vi "ex_Change Control Caption.vi"(4 "error in (no error)":errorcluster, 5 "New Name":string, 6 "Old Name":string, 7 "VI refnum":refnum<vi>) -> (0 "error out":errorcluster, 3 "Ctl refnum out":refnum<vi>)   [LabVIEW 2020]
doc: "Changes the label and the caption for a control specified by the control refnum on the VI specified by the VI refnum."
panel:
  in  "Ctl refnum":refnum<vi>
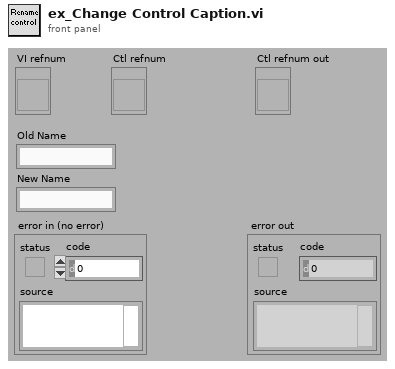
[diagram p1: front panel]
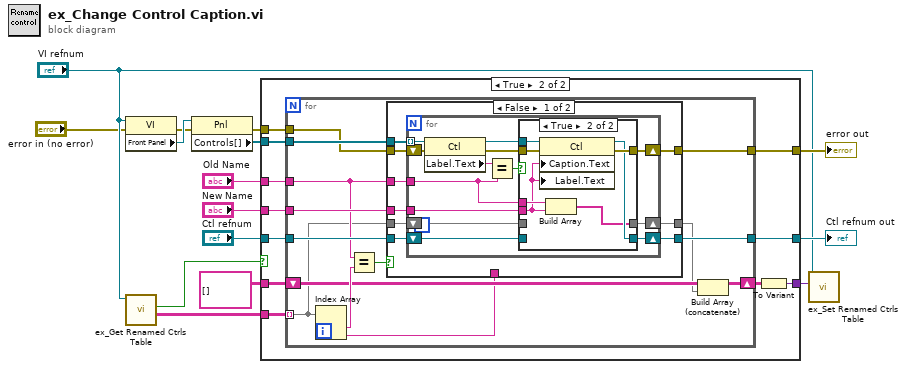
[diagram p0: block diagram]
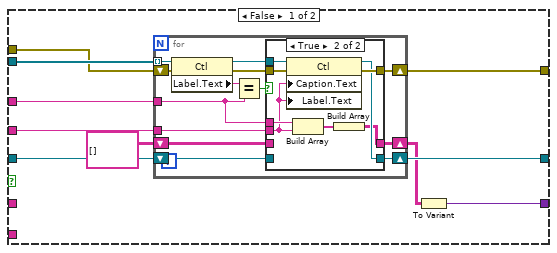
[diagram p2: hidden frame]
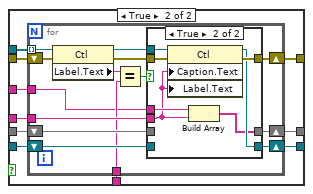
[diagram p5: hidden frame]
diagram:
  n1 = property class="VI"(reference="VI refnum", error in="error in (no error)") -> (error out=w11:errorcluster, "Front Panel"=w15:refnum<vi>)  [unwired: 1 out]
  n2 = call <vilib>:"ex_Get Renamed Ctrls Table.vi"("VI refnum"="VI refnum") -> ("Renamed Controls"=w1:string[][], "Tag available?"=w2:bool)  [unwired: 7 in, 2 out]
  n3 = property class="Pnl"(reference=w15, error in=w11) -> (error out=w9:errorcluster, "Controls[]"=w14:refnum<vi>[])  [unwired: 1 out]
  n4 = case shown="True" w2 {
    tunnel: w14 -> [w25 w59]
    tunnel: "Old Name" -> [w24 w55]
    tunnel: "New Name" -> [w23 w54]
    tunnel: [w22 w57] -> w10
    tunnel: w9 -> [w21 w53]
    tunnel: "Ctl refnum" -> [w20 w58]
    tunnel: [w19 w56] -> w7
    tunnel: w1 -> [_ w60]
    tunnel: [w16 w52] -> w6
    tunnel: string[][] [] ("Array") -> [_ w50]
    frame False {
      n5 = for {
        tunnel: w25 -> [w38] mode=indexing
        tunnel: w24 -> [w28]
        tunnel: w23 -> [w35]
        shift-right: [w32] -> w22
        shift-left: w21 -> [w31]
        shift-right: [w30] -> w19
        shift-left: w20 -> [w29]
        shift-right: [w27] -> w18
        shift-left: string[][] [] -> [w26]
        n6 = property class="Ctl"(reference=w38, error in=w31) -> (reference out=w36:refnum<vi>, error out=w33:errorcluster, "Label.Text"=w37:string)
        n7 = Equal?(x=w37, y=w28) -> (x = y?=w34:bool)
        n8 = case shown="True" w34 {
          tunnel: w36 -> [_ w49]
          tunnel: w35 -> [_ w44]
          tunnel: w33 -> [w41 w48]
          tunnel: [w41 w47] -> w32
          tunnel: [w40 w46] -> w30
          tunnel: w29 -> [w40 _]
          tunnel: w28 -> [_ w45]
          tunnel: [w39 w42] -> w27
          tunnel: w26 -> [w39 _]
          frame False {
          }
          frame True {
            n9 = property class="Ctl"(reference=w49, error in=w48, "Caption.Text"=w44, "Label.Text"=w44) -> (reference out=w46:refnum<vi>, error out=w47:errorcluster)
            n10 = Build Array(w45, w44) -> (w43:string[])
            n11 = Build Array(w43) -> (w42:string[][])
          }
        }
      }
      n12 = To Variant(anything=w18) -> (Variant=w16:variant)
    }
    frame True {
      n13 = for {
        tunnel: w60 -> [w62] mode=indexing
        tunnel: w59 -> [w74]
        tunnel: w58 -> [w73]
        tunnel: [w72] -> w57
        tunnel: [w71] -> w56
        tunnel: w55 -> [w67]
        tunnel: w54 -> [w70]
        tunnel: w53 -> [w69]
        shift-right: [w65] -> w51
        shift-left: w50 -> [w64]
        n14 = Index Array(array=w62) -> (element #1=w68:string, element #2=w61:string)  [unwired: 2 in]
        n15 = Equal?(x=w67, y=w68) -> (x = y?=w66:bool)
        n16 = case shown="False" w66 {
          tunnel: w74 -> [w83 w116]
          tunnel: w73 -> [w78 w115]
          tunnel: [w75 w114] -> w72
          tunnel: [w76 w113] -> w71
          tunnel: w70 -> [w80 w112]
          tunnel: w69 -> [w82 w111]
          tunnel: w67 -> [w81 w110]
          tunnel: [w77 w109] -> w63
          tunnel: w62 -> [w79 w108]
          tunnel: w61 -> [_ w107]
          frame False {
            n17 = for {
              tunnel: w83 -> [w96] mode=indexing
              tunnel: w81 -> [w86]
              tunnel: w80 -> [w93]
              shift-right: [w90] -> w75
              shift-left: w82 -> [w89]
              shift-right: [w88] -> w76
              shift-left: w78 -> [w87]
              shift-right: [w84] -> w77
              shift-left: w79 -> [w85]
              n18 = property class="Ctl"(reference=w96, error in=w89) -> (reference out=w94:refnum<vi>, error out=w91:errorcluster, "Label.Text"=w95:string)
              n19 = Equal?(x=w95, y=w86) -> (x = y?=w92:bool)
              n20 = case shown="True" w92 {
                tunnel: w94 -> [_ w106]
                tunnel: w93 -> [_ w101]
                tunnel: w91 -> [w99 w105]
                tunnel: [w99 w104] -> w90
                tunnel: [w98 w103] -> w88
                tunnel: w87 -> [w98 _]
                tunnel: w86 -> [_ w102]
                tunnel: [w97 w100] -> w84
                tunnel: w85 -> [w97 _]
                frame False {
                }
                frame True {
                  n21 = property class="Ctl"(reference=w106, error in=w105, "Caption.Text"=w101, "Label.Text"=w101) -> (reference out=w103:refnum<vi>, error out=w104:errorcluster)
                  n22 = Build Array(w102, w101) -> (w100:string[])
                }
              }
            }
          }
          frame True {
            n23 = for {
              tunnel: w116 -> [w130] mode=indexing
              tunnel: w110 -> [w117]
              tunnel: w112 -> [w127]
              shift-right: [w124] -> w114
              shift-left: w111 -> [w123]
              shift-right: [w122] -> w113
              shift-left: w115 -> [w121]
              shift-right: [w120] -> w109
              shift-left: w108 -> [w119]
              tunnel: w107 -> [w118]
              n24 = property class="Ctl"(reference=w130, error in=w123) -> (reference out=w128:refnum<vi>, error out=w125:errorcluster, "Label.Text"=w129:string)
              n25 = Equal?(x=w129, y=w118) -> (x = y?=w126:bool)
              n26 = case shown="True" w126 {
                tunnel: w128 -> [_ w140]
                tunnel: w127 -> [_ w135]
                tunnel: w125 -> [w133 w139]
                tunnel: [w133 w138] -> w124
                tunnel: [w132 w137] -> w122
                tunnel: w121 -> [w132 _]
                tunnel: w117 -> [_ w136]
                tunnel: [w131 w134] -> w120
                tunnel: w119 -> [w131 _]
                frame False {
                }
                frame True {
                  n27 = property class="Ctl"(reference=w140, error in=w139, "Caption.Text"=w135, "Label.Text"=w135) -> (reference out=w137:refnum<vi>, error out=w138:errorcluster)
                  n28 = Build Array(w136, w135) -> (w134:string[])
                }
              }
            }
          }
        }
        n29 = Build Array (concatenate)(w64, w63) -> (w65:string[][])
      }
      n30 = To Variant(anything=w51) -> (Variant=w52:variant)
    }
  }
  "error out" <- w10
  "Ctl refnum out" <- w7
  n31 = call <vilib>:"ex_Set Renamed Ctrls Table.vi"("Variant"=w6, "VI refnum"="VI refnum") -> ()  [unwired: 8 in, 2 out]
